vi "VISU_CRYO_FDS_LS218.vi"(0 "Port_COM":refnum<visa-resource-name>, 1 "table_acq":T2(array[cluster]), 2 "PÉRIODE ACQUISITION (sec)":i8(slide) scale=1.0..60.0, 3 "Nom manip":string, 4 "Celsius?":bool, 5 "error in (no error)":errorcluster caption="entrée d'erreur (pas d'erreur)", 8 "Répertoire":path) -> (14 "VISA_Out":refnum<visa-resource-name>, 19 "error out":errorcluster caption="sortie d'erreur")   [LabVIEW 2016]
uses:
  <vilib>/express/express signal manip/GetorSetDDTAttributes/Shared VIs/TimeType.ctl
  <vilib>/express/express signal manip/GetorSetDDTAttributes/Shared VIs/XDimension.ctl
  <vilib>/express/express signal manip/GetorSetDDTAttributes/Shared VIs/TimeMode Enum to Boolean.vi
  <vilib>/express/express signal manip/GetorSetDDTAttributes/Shared VIs/XDimension Enum to String.vi
  <vilib>/express/express shared/transition.llb/Dynamic To Waveform Array.vi
  <vilib>/express/express signal manip/GetorSetDDTAttributes/Set DDT Attributes/SetT0.vi
  <vilib>/express/express shared/transition.llb/Waveform Array To Dynamic.vi
  <vilib>/express/express signal manip/GetorSetDDTAttributes/Set DDT Attributes/Set DDT Properties.xnode
  <vilib>/express/express signal manip/GetorSetDDTAttributes/Shared VIs/GetSetShared.lvlib
panel:
  in  "Quitter":bool
  in  "Commande onglets":T1(tab)
  out "T_Glacon_C":dbl format="%#_5g °C"
  out "T_Glacon_K":dbl format="%#_g K"
  out "Mesures en cours":dynamicdata(graph)
  in  "Min/max fixes":bool
  in  "h":dbl min=0.0 max=24.0 format="%_1f"
  in  "min":dbl=1.0 min=0.0 max=59.0 format="%_1f"
  in  "Période fixe":bool
  in  "actualiser X":bool
  in  "Tmin\n (K)":dbl min=-273.0 max=1000.0 format="%#_3g"
  in  "Tmax\n (K)":dbl=300.0 min=-273.15 max=300.0 format="%#_3g"
  in  "actualiser Y":bool
  out "Température \nair liq C":dbl format="%#_5g °C"
  out "Température \nsortie°C":dbl format="%#_5g °C"
  out "Température \néchangeur °C":dbl format="%#_5g °C"
  out "Thermomètre":dbl(slide) min=-273.15 max=0.0 step=300.0 scale=-273.0..40.0
  out "Température\nair liquéfié":dbl format="%#_g K"
  out "Température\nsortie serpentin":dbl format="%#_g K"
  out "Température \néchangeur":dbl format="%#_g K"
  out "Échelle des X.Gamme:Début":dbl format="%<%H:%M:%S\n%x>T"
  out "Échelle des X.Gamme:Minimum":dbl format="%<%H:%M:%S\n%x>T"
  out "Échelle des X.Gamme:Maximum":dbl format="%<%H:%M:%S\n%x>T"
  out "taille_historique (s)":dbl
  out "Data_ligne":dbl[](array[numeric])
  in  "Vidange buffer":bool
  out "t_boucle_rec":i32
  out "Temps":u32
  out "Fichier d'acquisition":path
  out "Période (s)":i8
  out "Unité":string
  out "heure locale":timestamp
  out "heure début":timestamp
  # "J. HANSOTTE - IAS \nStation d'Étalonnage"
  # "CRYOGENIE"
  # "Glaçon plutonien !"
  # "Température"
  # "ÉCHELLE DE TEMPS"
  # "Auto"
  # "ÉCHELLE DE TEMPÉRATURE"
  # "Auto"
  # "L'alambic cryogénique : Liquéfaction du dioxygène"
  # "Air sec\nenv. 20°C"
  # "LO2"
  # "LN2"
  # "LN2"
  # "ÉCHANGEUR Air / LN2"
  # "Azote Liquide\n77K (-196°C)"
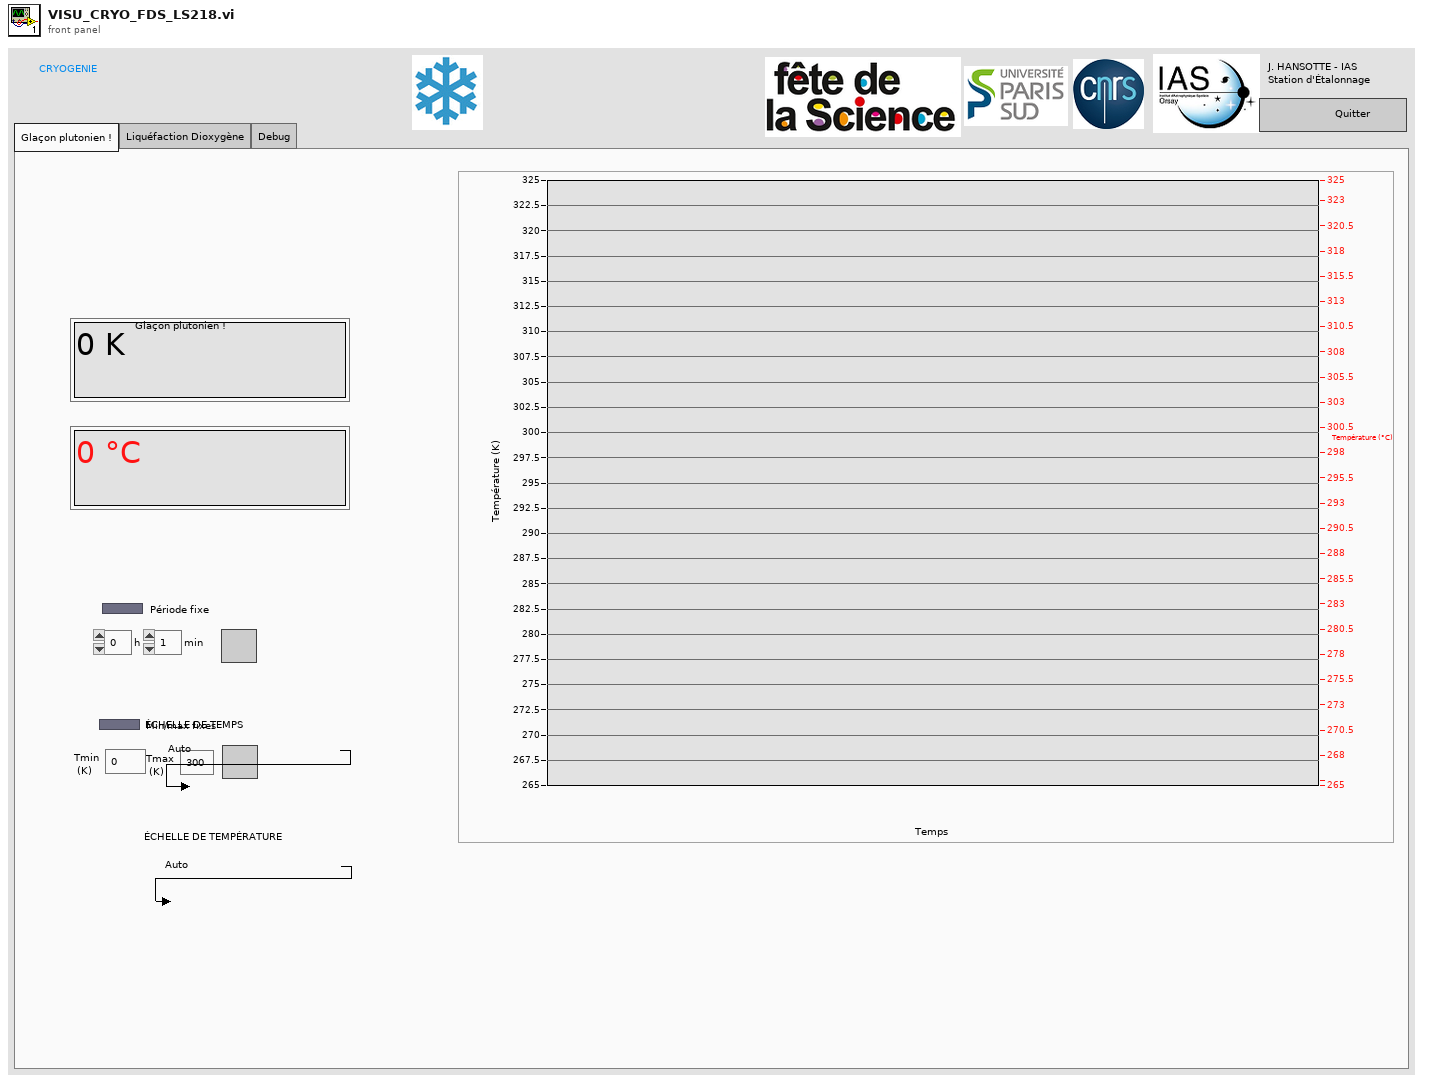
[diagram p1: front panel]
types:
  T1 = enum32{"Glaçon plutonien !", "Liquéfaction Dioxygène", "Debug"}
  T2 = cluster{"N_voie":i32, "Nom_voie":string, "Mesure_voie":dbl}[]
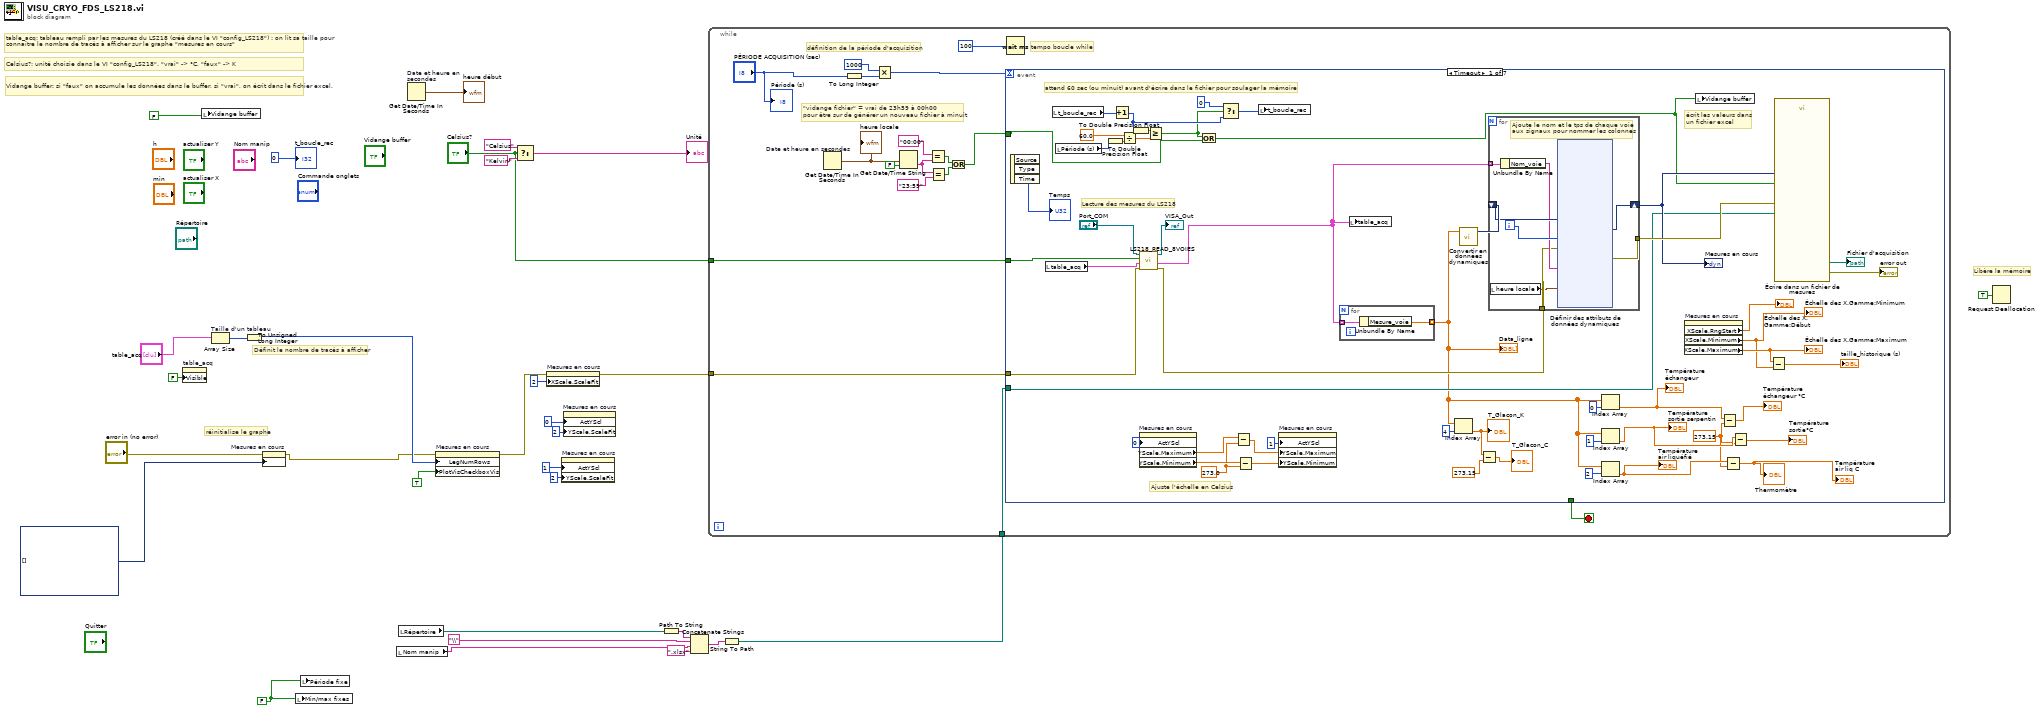
[diagram p0: block diagram]
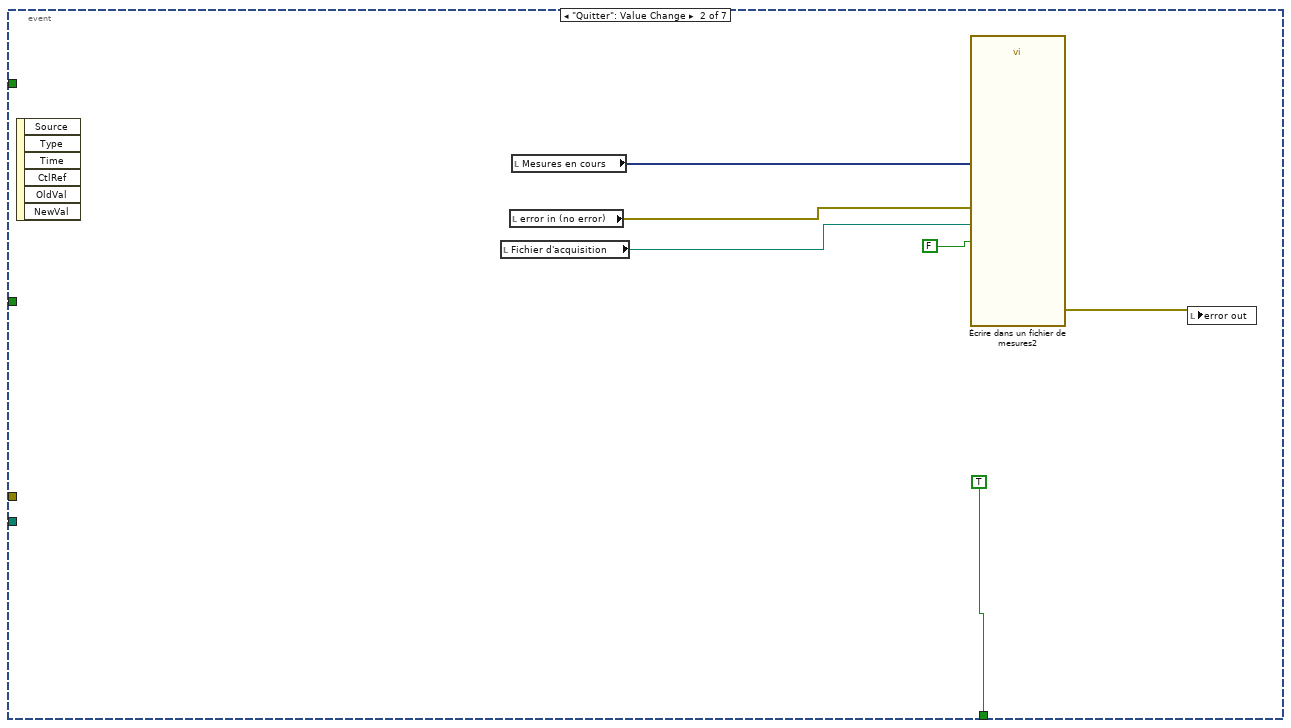
[diagram p2: hidden frame]
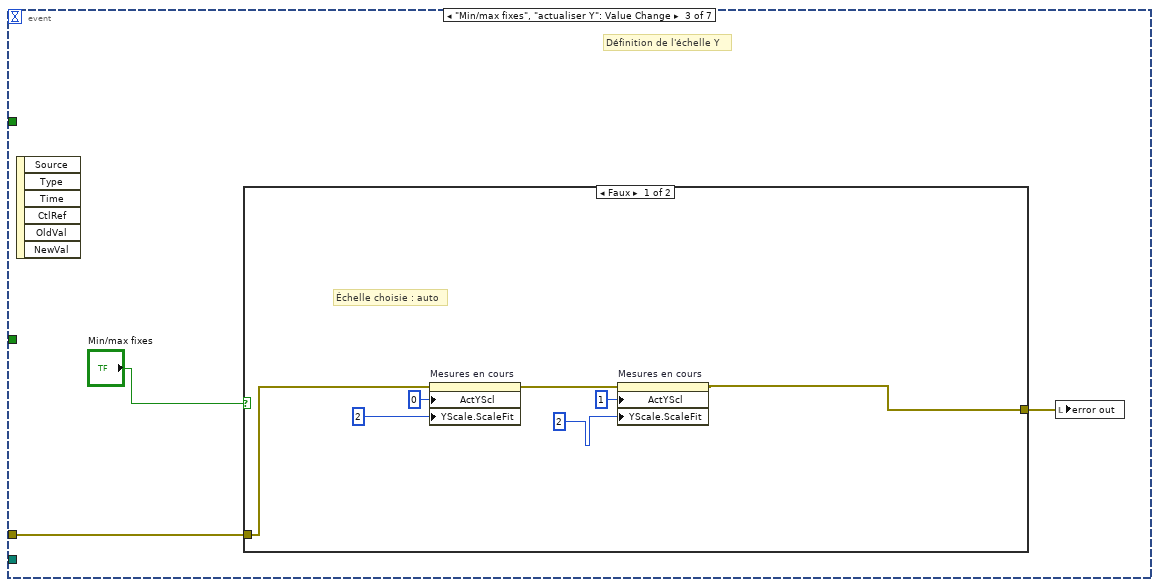
[diagram p3: hidden frame]
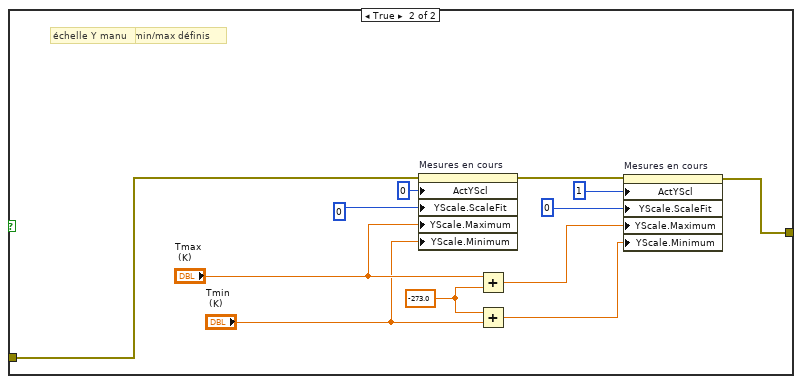
[diagram p4: hidden frame]
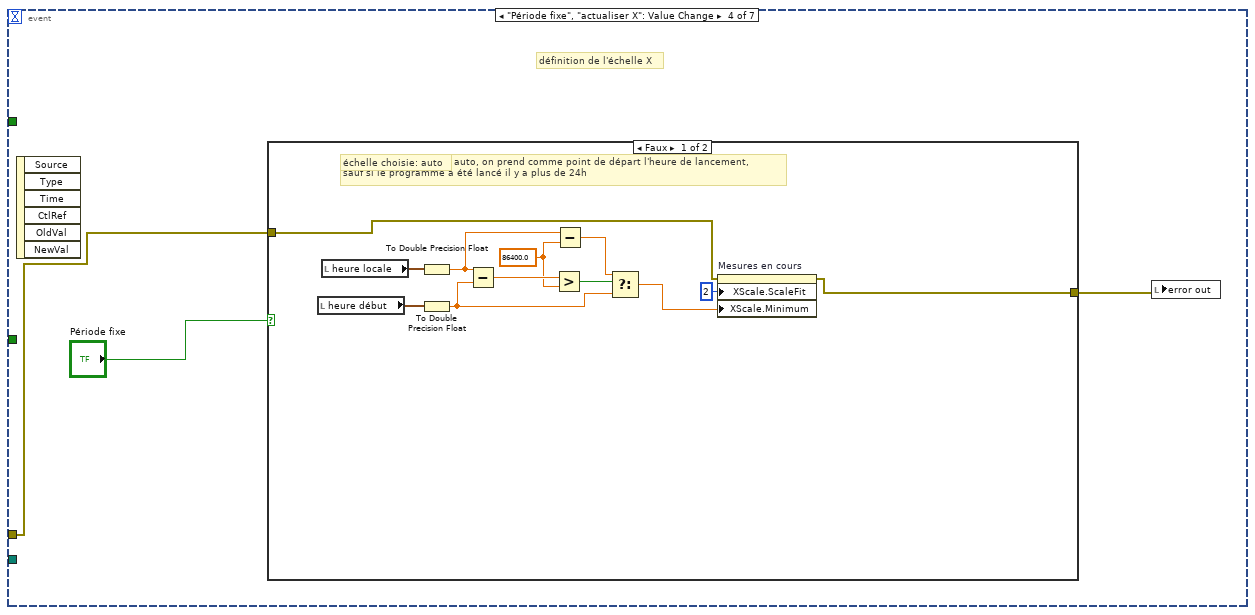
[diagram p5: hidden frame]
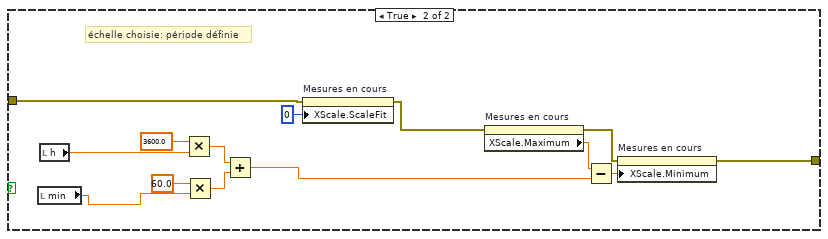
[diagram p6: hidden frame]
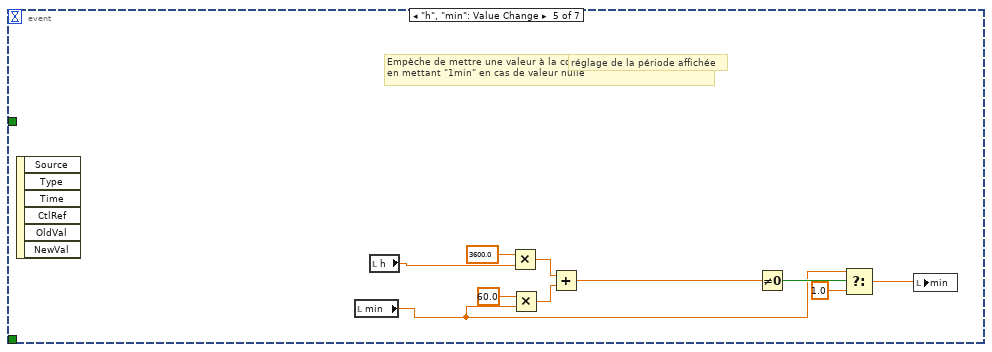
[diagram p7: hidden frame]
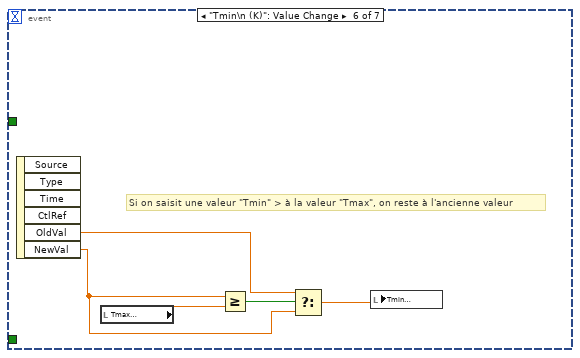
[diagram p8: hidden frame]
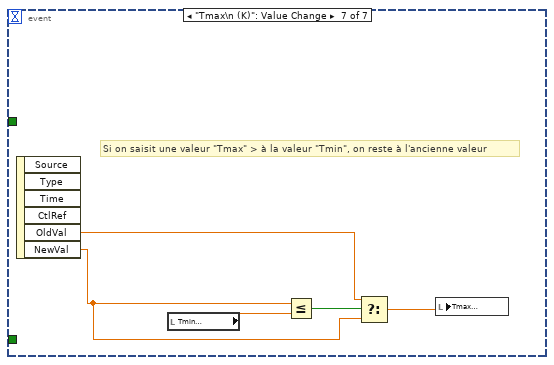
[diagram p9: hidden frame]
diagram:
  w18 = FALSE ("Visible")
  # "réinitialise le graphe"
  # "Vidange buffer: si \"faux\" on accumule les données dans le buffer, si \"vrai\", on écrit dans le fichier excel."
  # "Celsius?: unité choisie dans le VI \"config_LS218\". \"vrai\" -> °C, \"faux\" -> K"
  # "table_acq: tableau rempli par les mesures du LS218 (créé dans le VI \"config_LS218\") : on lit sa taille pour connaître le nombre de tracés à afficher sur le graphe \"mesures en cours\""
  # "Libère la mémoire"
  # "Définit le nombre de tracés à afficher"
  n1 = property on="table_acq" class="Tabl (strict)"("Visible"=FALSE) -> ()  [unwired: 2 in, 2 out]
  n2 = local write "Vidange buffer"(FALSE ("Vidange fichier temp")) -> ()
  n3 = Array Size "Taille d'un tableau"(array="table_acq") -> (size(s)=w28:i32)
  n4 = To Unsigned Long Integer(number=w28) -> (unsigned 32bit integer=w8:u32)
  n5 = property on="Mesures en cours" class="GraphDér (strict)"(error in="error in (no error)", "History Data"=dynamicdata[] [] ("Données d'historique")) -> (error out=w5:errorcluster)  [unwired: 1 in, 1 out]
  n6 = local write "Min/max fixes"(w18) -> ()
  n7 = local write "Période fixe"(w18) -> ()
  n8 = local read "Nom manip"() -> (w14:string)
  n9 = local read "Répertoire"() -> (w17:path)
  n10 = Get Date/Time In Seconds "Date et heure en secondes"() -> (seconds since 1Jan1904=→"heure début":timestamp)
  n11 = property on="Mesures en cours" class="GraphDér (strict)"(error in=w5, "LegNumRows"=w8, "PlotVisCheckboxVis"=TRUE ("Légende:Désactiver")) -> (error out=w9:errorcluster)  [unwired: 1 in, 1 out]
  n12 = Select(t="Celsius", s="Celsius?", f="Kelvin" ("cas faux")) -> (s? t:f=→"Unité":string)
  n13 = property on="Mesures en cours" class="GraphDér (strict)"(error in=w9, "XScale.ScaleFit"=u8 2 ("Échelle des X.Ajuster l'échelle")) -> (error out=w21:errorcluster)  [unwired: 1 in, 1 out]
  n14 = property on="Mesures en cours" class="GraphDér (strict)"("ActYScl"=u8 1 ("Échelle des Y.Ajuster l'échelle"), "YScale.ScaleFit"=u8 2 ("Échelle des Y.Ajuster l'échelle")) -> ()  [unwired: 2 in, 2 out]
  n15 = property on="Mesures en cours" class="GraphDér (strict)"("ActYScl"=u8 0 ("Échelle des Y.Ajuster l'échelle"), "YScale.ScaleFit"=u8 2 ("Échelle des Y.Ajuster l'échelle")) -> ()  [unwired: 2 in, 2 out]
  n16 = Path To String(path=w17) -> (string=w16:string)
  n17 = Concatenate Strings(w16, "\\" ("chaîne"), w14, ".xlsx" ("chaîne")) -> (w15:string)
  n18 = String To Path(string=w15) -> (path=w11:path)
  n19 = while {
    tunnel: "Celsius?" -> [w48]
    tunnel: w21 -> [w43]
    tunnel: w11 -> [w33]
    stop <- w32 stop-if-true
    # "\"vidange fichier\" = vrai de 23h59 à 00h00\npour être sur de générer un nouveau fichier à minuit"
    # "tempo boucle while"
    # "définition de la période d'acquisition"
    n20 = Get Date/Time In Seconds "Date et heure en secondes"() -> (seconds since 1Jan1904=w35:timestamp)
    "heure locale" <- w35
    n21 = To Long Integer(number="PÉRIODE ACQUISITION (sec)") -> (32bit integer=w46:i32)
    n22 = Multiply(x=1000, y=w46) -> (x*y=w44:i32)
    n23 = Get Date/Time String(seconds (now)=w35, want seconds? (F)=FALSE ("secondes ? (F)")) -> (time string=w40:string)  [unwired: 1 in, 1 out]
    n24 = Equal?(x="00:00", y=w40) -> (x = y?=w37:bool)
    n25 = Equal?(x=w40, y="23:59") -> (x = y?=w38:bool)
    n26 = Or(x=w37, y=w38) -> (x .or. y?=w36:bool)
    n27 = event shown="[0] Timeout" {
      selector: _ -> [_ _ _ _ _ _ _]
      dyn-events: _ -> [_ _ _ _ _ _ _]
      timeout: w44 -> [_ _ _ _ _ _ _]
      tunnel: w48 -> [w97 _ _ _ _ _ _]
      tunnel: w43 -> [w90 _ w146 w167 _ _ _]
      tunnel: w36 -> [w83 _ _ _ _ _ _]
      tunnel: w33 -> [w73 _ _ _ _ _ _]
      tunnel: [_ TRUE _ _ _ _ _] -> w32
      event Timeout {
        w49 = 273.0 ("y")
        w62 = 273.15 ("y")
        # "Ajuste l'échelle en Celsius"
        # "attend 60 sec (ou minuit) avant d'écrire dans le fichier pour soulager la mémoire"
        # "écrit les valeurs dans \nun fichier excel"
        # "Lecture des mesures du LS218"
        n28 = event-data() -> ("Time"=→"Temps":u32)  [unwired: 1 in, 2 out]
        n29 = local read "table_acq"() -> (w100:T2)
        n30 = local read "t_boucle_rec"() -> (w89:i32)
        n31 = local read "Période (s)"() -> (w77:i8)
        n32 = To Double Precision Float(number=w77) -> (double precision float=w75:dbl)
        n33 = Increment(x=w89) -> (x+1=w87:i32)
        n34 = Divide(x=60.0 ("y"), y=w75) -> (x/y=w76:dbl)
        n35 = To Double Precision Float(number=w87) -> (double precision float=w74:dbl)
        n36 = property on="Mesures en cours" class="GraphDér (strict)"("ActYScl"=0 ("Échelle active des Y")) -> ("YScale.Maximum"=w53:dbl, "YScale.Minimum"=w51:dbl)  [unwired: 2 in, 2 out]
        n37 = call "LS218_READ_8VOIES.vi"("entrée d'erreur (pas d'erreur)"=w90, "table_acq_in"=w100, "Celsius"=w97, "Refnum VISA en entrée"="Port_COM") -> ("sortie d'erreur"=w72:errorcluster, "table_acq_out"=w71:T2, "Nom de ressource VISA en sortie"=→"VISA_Out":refnum<visa-resource-name>)  [unwired: 1 in]
        n38 = Greater Or Equal?(x=w74, y=w76) -> (x >= y?=w85:bool)
        n39 = Or(x=w85, y=w83) -> (x .or. y?=w82:bool)
        n40 = Select(t=0 ("y"), s=w85, f=w87) -> (s? t:f=w86:i32)
        n41 = Subtract(x=w53, y=w49) -> (x-y=w52:dbl)
        n42 = Subtract(x=w51, y=w49) -> (x-y=w50:dbl)
        n43 = local write "t_boucle_rec"(w86) -> ()
        n44 = property on="Mesures en cours" class="GraphDér (strict)"("ActYScl"=1 ("Échelle active des Y"), "YScale.Maximum"=w52, "YScale.Minimum"=w50) -> ()  [unwired: 2 in, 2 out]
        n45 = for {
          tunnel: w71 -> [w137] mode=indexing
          tunnel: [w136] -> w59 mode=indexing
          n46 = Unbundle By Name(w137) -> ("Mesure_voie"=w136:dbl)
        }
        "Data_ligne" <- w59
        n47 = local write "table_acq"(w71) -> ()
        n48 = Index Array(array=w59, index=4 ("indice")) -> (element=w58:dbl)
        "T_Glacon_K" <- w58
        n49 = call "Convertir en données dynamiques"("Array"=w59) -> ("Dynamic Data Type"=w93:dynamicdata)  [unwired: 3 in]
        n50 = Subtract(x=w58, y=273.15) -> (x-y=→"T_Glacon_C":dbl)
        n51 = for {
          shift-right: [w107] -> w91
          shift-left: w93 -> [w108]
          tunnel: w71 -> [w105] mode=indexing
          tunnel: w72 -> [w103]
          tunnel: [w102] -> w92
          i -> [w106]
          # "Ajoute le nom et le tps de chaque voie\naux signaux pour nommer les colonnes"
          n52 = local read "heure locale"() -> (w101:timestamp)
          n53 = Unbundle By Name(w105) -> ("Nom_voie"=w104:string)
          n54 = xnode "Définir des attributs de données dynamiques"("Signaux en entrée"=w108, "Indice du signal"=w106, "entrée d'erreur"=w103, "Nom du signal"=w104, "Horodatage"=w101) -> ("Signaux en sortie"=w107:dynamicdata, "sortie d'erreur"=w102:errorcluster)  [unwired: 2 in]
        }
        "Mesures en cours" <- w91
        n55 = Index Array(array=w59, index=0 ("indice")) -> (element=w67:dbl)
        "Température \néchangeur" <- w67
        n56 = Index Array(array=w59, index=1 ("indice")) -> (element=w64:dbl)
        "Température\nsortie serpentin" <- w64
        n57 = Index Array(array=w59, index=2 ("indice")) -> (element=w63:dbl)
        "Température\nair liquéfié" <- w63
        n58 = property on="Mesures en cours" class="GraphDér (strict)"() -> ("XScale.RngStart"=→"Échelle des X.Gamme:Début":dbl, "XScale.Minimum"=w80:dbl, "XScale.Maximum"=w81:dbl)  [unwired: 2 in, 2 out]
        "Échelle des X.Gamme:Minimum" <- w80
        "Échelle des X.Gamme:Maximum" <- w81
        n59 = local write "Vidange buffer"(w82) -> ()
        n60 = Subtract(x=w67, y=w62) -> (x-y=→"Température \néchangeur °C":dbl)
        n61 = Subtract(x=w63, y=w62) -> (x-y=→"Thermomètre" →"Température \nair liq C":dbl)
        n62 = Subtract(x=w64, y=w62) -> (x-y=→"Température \nsortie°C":dbl)
        n63 = Subtract(x=w81, y=w80) -> (x-y=→"taille_historique (s)":dbl)
        n64 = call "Écrire dans un fichier de mesures"("Signals"=w91, "Flush? (T)"=w82, "error in (no error)"=w92, "Filename"=w73) -> ("Filename Out"=→"Fichier d'acquisition":path, "error out"=→"error out":errorcluster)  [unwired: 13 in, 1 out]
      }
      event "Quitter": Value Change {
        n65 = event-data() -> ()  [unwired: 1 in, 6 out]
        n66 = local read "Fichier d'acquisition"() -> (w142:path)
        n67 = local read "error in (no error)"() -> (w141:errorcluster)
        n68 = local read "Mesures en cours"() -> (w143:dynamicdata)
        n69 = call "Écrire dans un fichier de mesures2"("Signals"=w143, "Reset"=FALSE, "error in (no error)"=w141, "Filename"=w142) -> ("error out"=w140:errorcluster)  [unwired: 13 in, 2 out]
        n70 = local write "error out"(w140) -> ()
      }
      event "Min/max fixes", "actualiser Y": Value Change {
        # "Définition de l'échelle Y"
        n71 = event-data() -> ()  [unwired: 1 in, 6 out]
        n72 = case shown="Faux" "Min/max fixes" {
          tunnel: w146 -> [w153 w165]
          tunnel: [w147 w161] -> w145
          frame False {
            # "Échelle choisie : auto"
            n73 = property on="Mesures en cours" class="GraphDér (strict)"(error in=w153, "ActYScl"=0 ("Échelle active des Y"), "YScale.ScaleFit"=u8 2 ("cas vrai")) -> (error out=w152:errorcluster)  [unwired: 1 in, 1 out]
            n74 = property on="Mesures en cours" class="GraphDér (strict)"(error in=w152, "ActYScl"=1 ("Échelle active des Y"), "YScale.ScaleFit"=u8 2 ("Échelle des Y.Ajuster l'échelle")) -> (error out=w147:errorcluster)  [unwired: 1 in, 1 out]
          }
          frame True {
            w154 = -273.0 ("y")
            # "Échelle choisie : min/max définis"
            # "échelle Y manu"
            n75 = property on="Mesures en cours" class="GraphDér (strict)"(error in=w165, "ActYScl"=0 ("Échelle active des Y"), "YScale.ScaleFit"=u8 0 ("cas faux"), "YScale.Maximum"="Tmax\n (K)", "YScale.Minimum"="Tmin\n (K)") -> (error out=w162:errorcluster)  [unwired: 1 in, 1 out]
            n76 = Add(x="Tmax\n (K)", y=w154) -> (x+y=w157:dbl)
            n77 = Add(x=w154, y="Tmin\n (K)") -> (x+y=w155:dbl)
            n78 = property on="Mesures en cours" class="GraphDér (strict)"(error in=w162, "ActYScl"=1 ("Échelle active des Y"), "YScale.ScaleFit"=u8 0 ("cas faux"), "YScale.Maximum"=w157, "YScale.Minimum"=w155) -> (error out=w161:errorcluster)  [unwired: 1 in, 1 out]
          }
        }
        n79 = local write "error out"(w145) -> ()
      }
      event "Période fixe", "actualiser X": Value Change {
        # "définition de l'échelle X"
        n80 = event-data() -> ()  [unwired: 1 in, 6 out]
        n81 = case shown="Faux" "Période fixe" {
          tunnel: w167 -> [w169 w184]
          tunnel: [w170 w181] -> w166
          frame False {
            w174 = 86400.0 ("y")
            # "échelle choisie: auto"
            # "Au passage en échelle auto, on prend comme point de départ l'heure de lancement,\nsauf si le programme a été lancé il y a plus de 24h"
            n82 = local read "heure début"() -> (w179:timestamp)
            n83 = local read "heure locale"() -> (w173:timestamp)
            n84 = To Double Precision Float(number=w173) -> (double precision float=w172:dbl)
            n85 = To Double Precision Float(number=w179) -> (double precision float=w175:dbl)
            n86 = Subtract(x=w172, y=w175) -> (x-y=w178:dbl)
            n87 = Greater?(x=w178, y=w174) -> (0:w177:bool)
            n88 = Subtract(x=w172, y=w174) -> (x-y=w171:dbl)
            n89 = Select(t=w171, s=w177, f=w175) -> (s? t:f=w176:dbl)
            n90 = property on="Mesures en cours" class="GraphDér (strict)"(error in=w169, "XScale.ScaleFit"=u8 2 ("Échelle des X.Ajuster l'échelle"), "XScale.Minimum"=w176) -> (error out=w170:errorcluster)  [unwired: 1 in, 1 out]
          }
          frame True {
            # "échelle choisie: période définie"
            n91 = local read "min"() -> (w187:dbl)
            n92 = local read "h"() -> (w186:dbl)
            n93 = Multiply(x=3600.0, y=w186) -> (x*y=w193:dbl)
            n94 = Multiply(x=60.0, y=w187) -> (x*y=w194:dbl)
            n95 = Add(x=w193, y=w194) -> (x+y=w188:dbl)
            n96 = property on="Mesures en cours" class="GraphDér (strict)"(error in=w184, "XScale.ScaleFit"=u8 0 ("Échelle des X.Ajuster l'échelle")) -> (error out=w183:errorcluster)  [unwired: 1 in, 1 out]
            n97 = property on="Mesures en cours" class="GraphDér (strict)"(error in=w183) -> (error out=w182:errorcluster, "XScale.Maximum"=w189:dbl)  [unwired: 1 in, 1 out]
            n98 = Subtract(x=w189, y=w188) -> (x-y=w190:dbl)
            n99 = property on="Mesures en cours" class="GraphDér (strict)"(error in=w182, "XScale.Minimum"=w190) -> (error out=w181:errorcluster)  [unwired: 1 in, 1 out]
          }
        }
        n100 = local write "error out"(w166) -> ()
      }
      event "h", "min": Value Change {
        # "réglage de la période affichée"
        # "Empèche de mettre une valeur à la con (temps nul ou négatif)\nen mettant \"1min\" en cas de valeur nulle"
        n101 = event-data() -> ()  [unwired: 1 in, 6 out]
        n102 = local read "min"() -> (w195:dbl)
        n103 = local read "h"() -> (w200:dbl)
        n104 = Multiply(x=3600.0, y=w200) -> (x*y=w203:dbl)
        n105 = Multiply(x=60.0, y=w195) -> (x*y=w204:dbl)
        n106 = Add(x=w203, y=w204) -> (x+y=w199:dbl)
        n107 = Not Equal To 0?(x=w199) -> (x != 0?=w198:bool)
        n108 = Select(t=w195, s=w198, f=1.0 ("cas faux")) -> (s? t:f=w196:dbl)
        n109 = local write "min"(w196) -> ()
      }
      event "Tmin\n (K)": Value Change {
        # "Si on saisit une valeur \"Tmin\" > à la valeur \"Tmax\", on reste à l'ancienne valeur"
        n110 = event-data() -> ("OldVal"=w207:dbl, "NewVal"=w206:dbl)  [unwired: 1 in, 4 out]
        n111 = local read "Tmax\n (K)"() -> (w209:dbl)
        n112 = Greater Or Equal?(x=w206, y=w209) -> (x >= y?=w208:bool)
        n113 = Select(t=w207, s=w208, f=w206) -> (s? t:f=w205:dbl)
        n114 = local write "Tmin\n (K)"(w205) -> ()
      }
      event "Tmax\n (K)": Value Change {
        # "Si on saisit une valeur \"Tmax\" > à la valeur \"Tmin\", on reste à l'ancienne valeur"
        n115 = event-data() -> ("OldVal"=w211:dbl, "NewVal"=w210:dbl)  [unwired: 1 in, 4 out]
        n116 = local read "Tmin\n (K)"() -> (w214:dbl)
        n117 = Less Or Equal?(x=w210, y=w214) -> (x <= y?=w213:bool)
        n118 = Select(t=w211, s=w213, f=w210) -> (s? t:f=w212:dbl)
        n119 = local write "Tmax\n (K)"(w212) -> ()
      }
    }
    n120 = Wait (ms)(milliseconds to wait=u32 100 ("attente (ms)")) -> ()  [unwired: 1 out]
    "Période (s)" <- "PÉRIODE ACQUISITION (sec)"
  }
  n121 = Request Deallocation(TRUE ("flag")) -> ()
  "t_boucle_rec" <- 0 ("t_boucle_rec")
